vi "DC Precharge Test TSFTS2.vi"(8 "error in (no error)":errorcluster) -> (0 "error out":errorcluster, 1 "Result (bool)":bool, 3 "VISA Refnum out":refnum<visa-resource-name>)   [LabVIEW 2022 SP3]
panel:
  in  "Bypass":bool
  in  "stop":bool
  out "Instructional Message":string
  in  "OK Button":bool
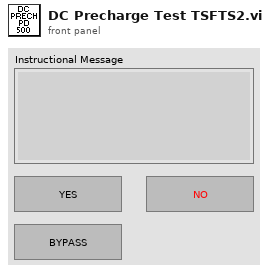
[diagram p1: front panel]
types:
  T1 = cluster{"Relay Command":bool[], "Inst. Message":string}[]
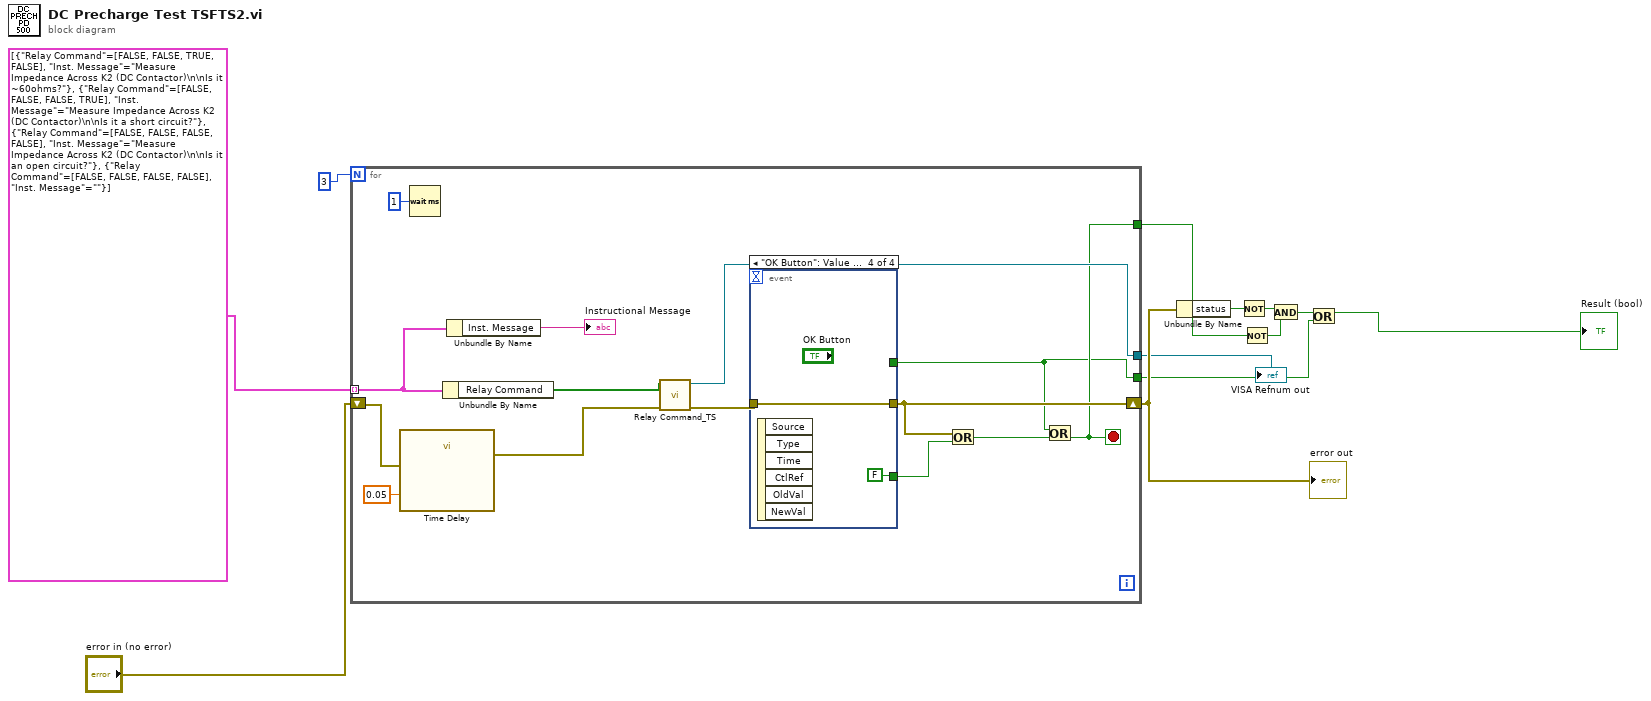
[diagram p0: block diagram]
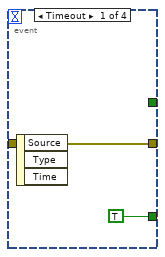
[diagram p2: hidden frame]
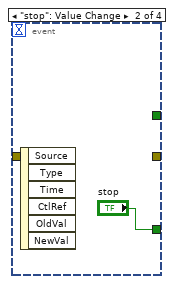
[diagram p3: hidden frame]
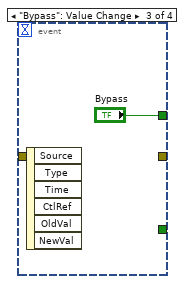
[diagram p4: hidden frame]
diagram:
  n1 = for {
    N: 3 -> [_]
    shift-right: [w26] -> w10
    shift-left: "error in (no error)" -> [w17]
    tunnel: T1 [{"Relay Command"=[FALSE, FALSE, TRUE, FALSE], "Inst. Message"="Measure Impedance Across K2 (DC Contactor)\n\nIs it ~60ohms?"}, {"Relay Command"=[FALSE, FALSE, FALSE, TRUE], "Inst. Message"="Measure Impedance Across K2 (DC Contactor)\n\nIs it a short circuit?"}, {"Relay Command"=[FALSE, FALSE, FALSE, FALSE], "Inst. Message"="Measure Impedance Across K2 (DC Contactor)\n\nIs it an open circuit?"}, {"Relay Command"=[FALSE, FALSE, FALSE, FALSE], "Inst. Message"=""}] -> [w24] mode=indexing
    tunnel: [w19] -> w2
    tunnel: [w20] -> w7
    tunnel: [w18] -> w3
    stop <- w19 stop-if-true
    n2 = call "Time Delay"("error in (no error)"=w17, "Delay Time (s)"=0.05) -> ("error out"=w16:errorcluster)  [unwired: 9 in]
    n3 = Wait (ms)(milliseconds to wait=u32 1) -> ()  [unwired: 1 out]
    n4 = Unbundle By Name(w24) -> ("Relay Command"=w14:bool[])
    n5 = Unbundle By Name(w24) -> ("Inst. Message"=→"Instructional Message":string)
    n6 = call "Relay Command_TS.vi"("error in (no error)"=w16, "Relay Command"=w14) -> ("error out"=w21:errorcluster, "VISA Refnum out"=w20:refnum<visa-resource-name>)  [unwired: 8 in]
    n7 = event shown="[3] \"OK Button\": Value Change" {
      selector: _ -> [_ _ _ _]
      dyn-events: _ -> [_ _ _ _]
      timeout: _ -> [_ _ _ _]
      tunnel: w21 -> [w28 _ _ w32]
      tunnel: [w28 _ _ w32] -> w26
      tunnel: [TRUE "stop" _ FALSE] -> w23
      tunnel: [_ _ "Bypass" _] -> w18
      event Timeout {
        n8 = event-data() -> ()  [unwired: 1 in, 3 out]
      }
      event "stop": Value Change {
        n9 = event-data() -> ()  [unwired: 1 in, 6 out]
      }
      event "Bypass": Value Change {
        n10 = event-data() -> ()  [unwired: 1 in, 6 out]
      }
      event "OK Button": Value Change {
        n11 = event-data() -> ()  [unwired: 1 in, 6 out]
      }
    }
    n12 = Or(x=w26, y=w23) -> (x .or. y?=w22:bool)
    n13 = Or(x=w18, y=w22) -> (x .or. y?=w19:bool)
  }
  "error out" <- w10
  "VISA Refnum out" <- w7
  n14 = Unbundle By Name(w10) -> ("status"=w12:bool)
  n15 = Not(x=w12) -> (.not. x?=w11:bool)
  n16 = Not(x=w2) -> (.not. x?=w8:bool)
  n17 = And(x=w11, y=w8) -> (x .and. y?=w5:bool)
  n18 = Or(x=w5, y=w3) -> (x .or. y?=→"Result (bool)":bool)
